vi "Init Outgoing Cyclic Signals.vi"(8 "error in":errorcluster, 11 "Outgoing Cyclic Configuraiton":T1 {"Outgoing Cyclic Frame"."Transmit Propreties"."Transmit Time" format="%#_p"}) -> (0 "error out":errorcluster, 3 "Outgoing Cyclic Configuraiton":T5 {"Outgoing Cyclic Frame"."Transmit Propreties"."Transmit Time" format="%#_p"})   [LabVIEW 2015, in "J1939 Addon Engine.lvlib"]
uses:
  J1939 Addon Engine.lvlib
  Types/Outgoing Cyclic Configuration.ctl
  Types/Outgoing Cyclic Frame Pairs.ctl
  Shared/Types/XNET Frame Event Properties.ctl
  Shared/Types/Outgoing Cyclic Channel Pairs.ctl
  Shared/Types/SysDef Outgoing Cyclic Configurations.ctl
  Shared/Types/SysDef Outgoing Frame Configuration.ctl
  <vilib>/xnet/xnet.llb/XNET Create Session (Conversion).vi
  Shared/J1939 Addon Shared.lvlib
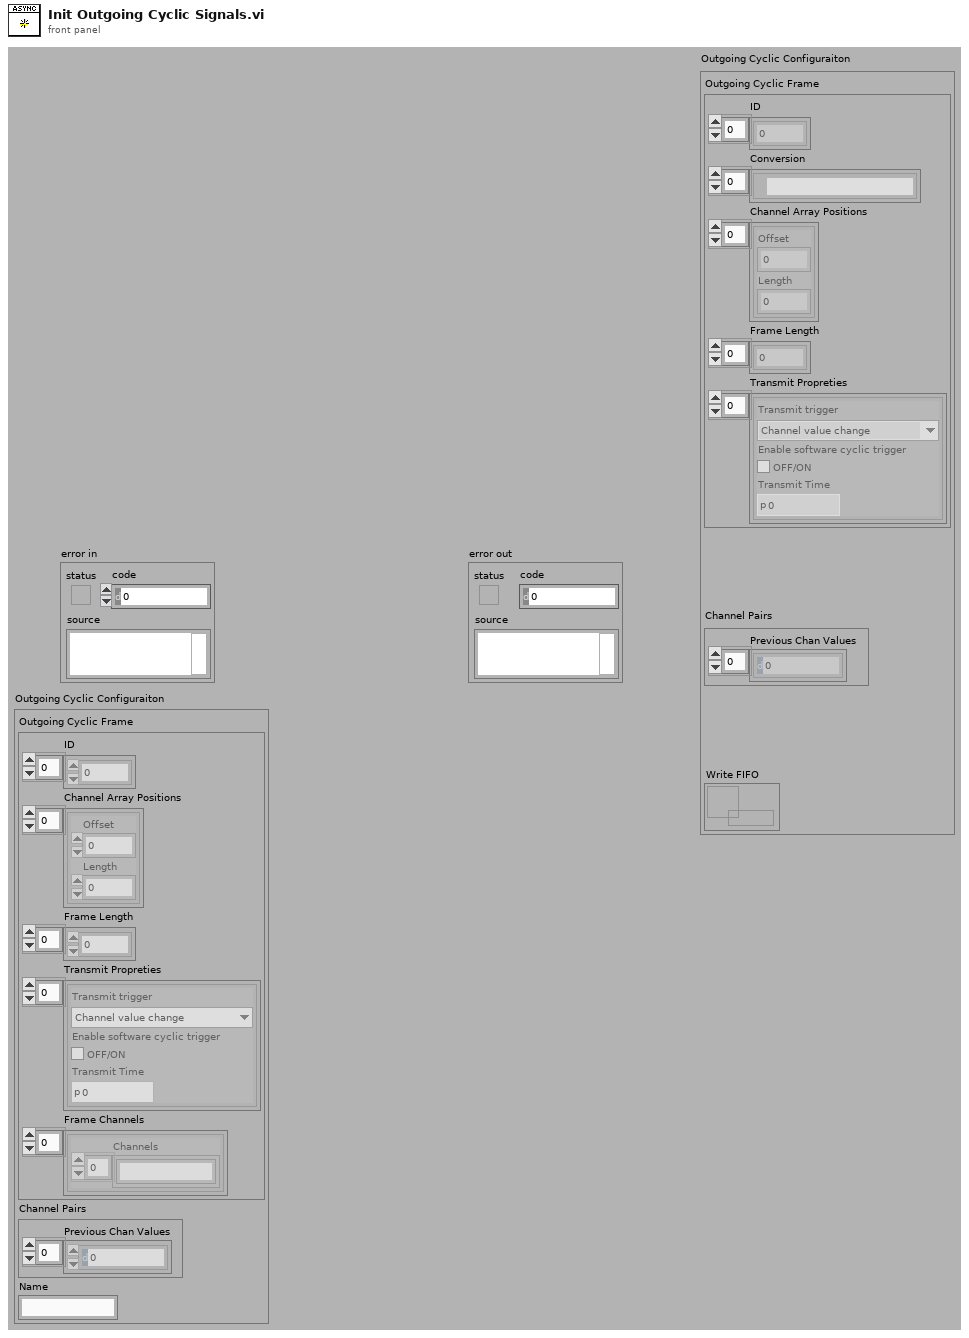
[diagram p1: front panel]
types:
  T1 = typedef "J1939 Addon Shared.lvlib/SysDef Outgoing Cyclic Configurations.ctl" = cluster{"Outgoing Cyclic Frame":T2, "Channel Pairs":T4, "Name":string}
  T2 = typedef "J1939 Addon Shared.lvlib/SysDef Outgoing Frame Configuration.ctl" = cluster{"ID":u32[], "Channel Array Positions":cluster{"Offset":u32, "Length":u32}[], "Frame Length":u32[], "Transmit Propreties":T3[], "Frame Channels":cluster{"Channels":string[]}[]}
  T3 = typedef "J1939 Addon Shared.lvlib/XNET Frame Event Properties.ctl" = cluster{"Transmit trigger":enum16{"Channel value change"}, "Enable software cyclic trigger":bool, "Transmit Time":dbl}
  T4 = typedef "J1939 Addon Shared.lvlib/Outgoing Cyclic Channel Pairs.ctl" = cluster{"Previous Chan Values":dbl[]}
  T5 = typedef "J1939 Addon Engine.lvlib/Outgoing Cyclic Configuration.ctl" = cluster{"Outgoing Cyclic Frame":T6, "Channel Pairs":T4, "Write FIFO":refnum<k33>}
  T6 = typedef "J1939 Addon Engine.lvlib/Outgoing Cyclic Frame Pairs.ctl" = cluster{"ID":u32[], "Conversion":refnum<k21>[], "Channel Array Positions":cluster{"Offset":u32, "Length":u32}[], "Frame Length":u32[], "Transmit Propreties":T3[]}
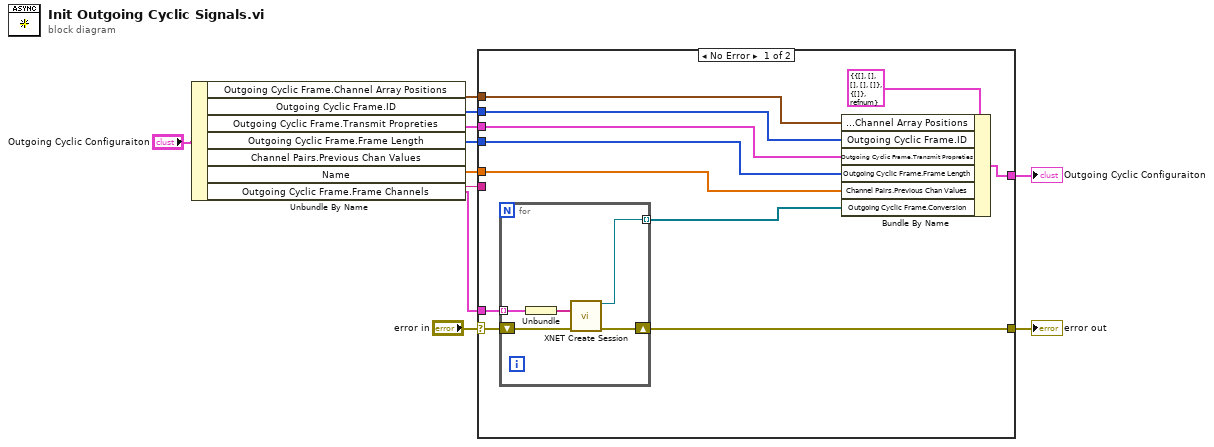
[diagram p0: block diagram]
diagram:
  n1 = Unbundle By Name("Outgoing Cyclic Configuraiton") -> ("Outgoing Cyclic Frame.Channel Array Positions"=w3:cluster{"Offset":u32, "Length":u32}[], "Outgoing Cyclic Frame.ID"=w2:u32[], "Outgoing Cyclic Frame.Transmit Propreties"=w4:T3[], "Outgoing Cyclic Frame.Frame Length"=w5:u32[], "Channel Pairs.Previous Chan Values"=w6:dbl[], "Name"=w1:string, "Outgoing Cyclic Frame.Frame Channels"=w7:cluster{"Channels":string[]}[])
  n2 = case shown="No Error" "error in" {
    selector: "error in" -> [w18 w28]
    tunnel: [w22 _] -> w9
    tunnel: [w12 w28] -> w11
    tunnel: w7 -> [w20 _]
    tunnel: w6 -> [w19 _]
    tunnel: w5 -> [w16 _]
    tunnel: w4 -> [w15 _]
    tunnel: w3 -> [w14 _]
    tunnel: w2 -> [w13 _]
    tunnel: w1 -> [_ _]
    frame No Error {
      n3 = for {
        shift-right: [w27] -> w12
        shift-left: w18 -> [w23]
        tunnel: [w26] -> w17 mode=indexing
        tunnel: w20 -> [w25] mode=indexing
        n4 = Unbundle(w25) -> ("Channels"=w24:string[])
        n5 = call-poly <vilib>:"XNET Create Session.vi"("signal list"=w24, "error in (no error)"=w23) -> ("session out"=w26:refnum<k21>, "error out"=w27:errorcluster)  [unwired: 12 in]
      }
      n6 = Bundle By Name(cluster=T5 {"Outgoing Cyclic Frame"={"ID"=[], "Conversion"=[], "Channel Array Positions"=[], "Frame Length"=[], "Transmit Propreties"=[]}, "Channel Pairs"={"Previous Chan Values"=[]}, "Write FIFO"=refnum} ("Outgoing Cyclic Configuraiton"), "Outgoing Cyclic Frame.Channel Array Positions"=w14, "Outgoing Cyclic Frame.ID"=w13, "Outgoing Cyclic Frame.Transmit Propreties"=w15, "Outgoing Cyclic Frame.Frame Length"=w16, "Channel Pairs.Previous Chan Values"=w19, "Outgoing Cyclic Frame.Conversion"=w17) -> (w22:T5)
    }
    frame Error {
    }
  }
  "error out" <- w11
  "Outgoing Cyclic Configuraiton" <- w9
